vi "ACal-Create Weighted Stimulus.vi"(0 "Weighted":T3 {"WF" items=["Chirp", "Noise"]}, 5 "Cal Stimulus":T1, 7 "Speaker":T2, 11 "error in (no error)":errorcluster) -> (4 "Stimulus":dbl[](array[numeric]), 15 "error out":errorcluster)   [LabVIEW 2020]
uses:
  Type Defs/ACal-Multiband Parameters.ctl
  epl-vi-lib/Utility VIs/Type Defs/Speaker ring.ctl
  Type Defs/Cal Stimulus.ctl
  Inverse Filter VIs/InvFilt-Params.ctl
  epl-vi-lib/Utility VIs/Math VIs/dB to Linear (scalar).vi
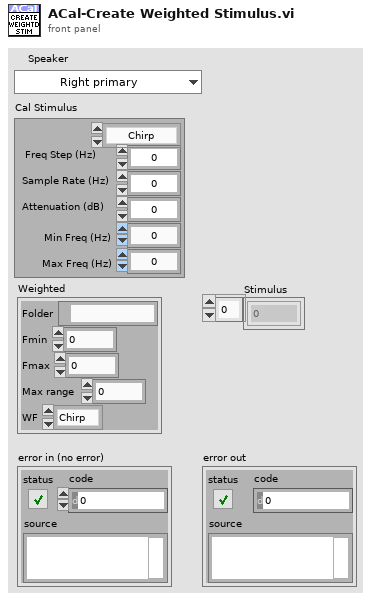
[diagram p1: front panel]
types:
  T1 = typedef "Cal Stimulus.ctl" = cluster{"Min Freq (Hz)":dbl, "Max Freq (Hz)":dbl, "Freq Step (Hz)":dbl, "Waveform":enum16{"Chirp", "Weighted"}, "Attenuation (dB)":dbl, "Sample Rate (Hz)":dbl}
  T2 = typedef "Speaker ring.ctl" = enum16{"Right primary", "Right secondary", "Left primary", "Left secondary"}
  T3 = typedef "ACal-Multiband Parameters.ctl" = cluster{"Folder":path, "Fmin":dbl, "Fmax":dbl, "Max range":dbl, "WF":u16}
  T4 = typedef "InvFilt-Params.ctl" = cluster{"Min Frequency (Hz)":dbl, "Max Frequency (Hz)":dbl, "Length (points)":i32, "Sampling rate (Hz)":dbl, "Delay (ms)":dbl, "Linear phase":bool}
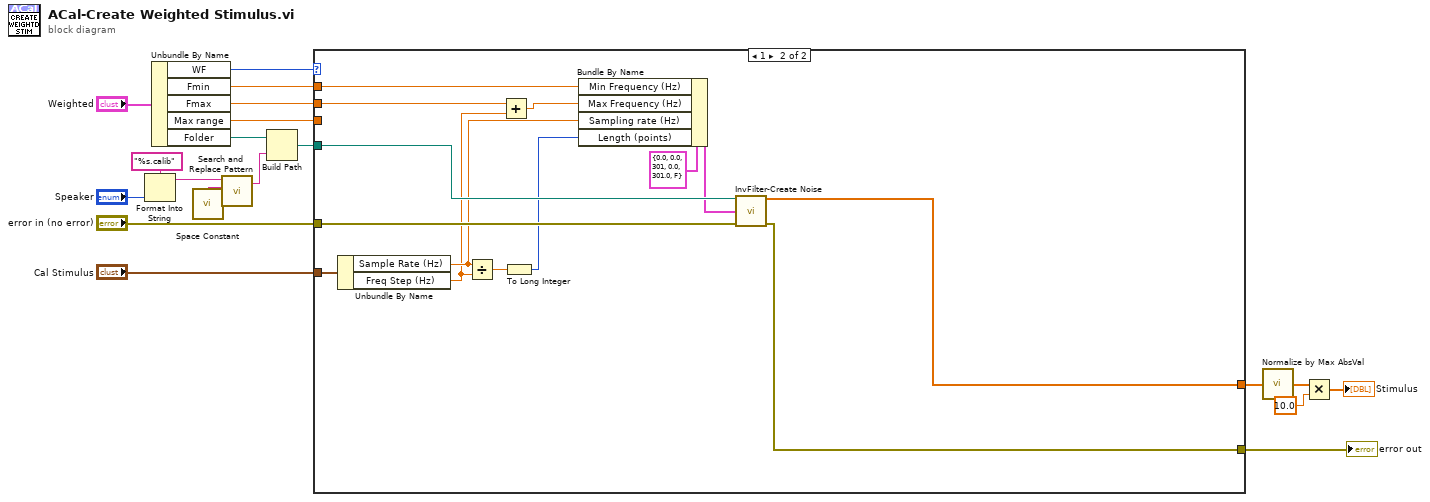
[diagram p0: block diagram]
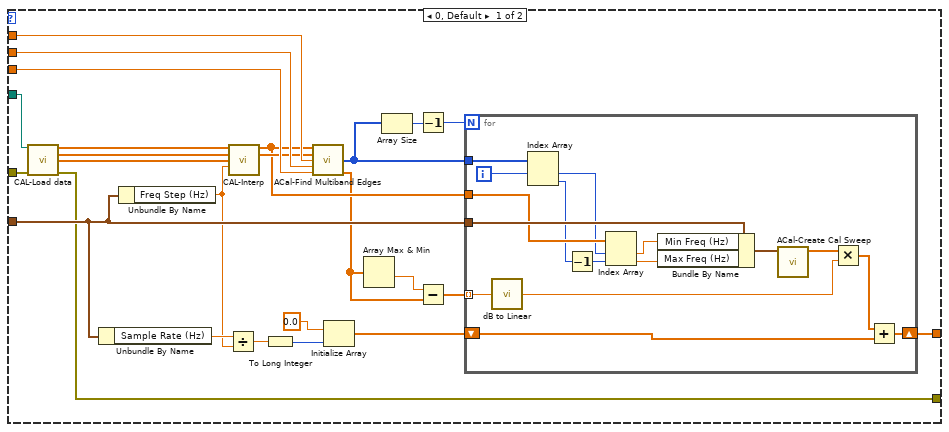
[diagram p2: hidden frame]
diagram:
  n1 = Format Into String(format string="%s.calib", "Speaker") -> (resulting string=w9:string)  [unwired: 2 in, 1 out]
  n2 = Unbundle By Name("Weighted") -> ("WF"=w5:u16, "Fmin"=w12:dbl, "Fmax"=w13:dbl, "Max range"=w14:dbl, "Folder"=w18:path)
  n3 = call <vilib>:"Space Constant.vi"() -> ("String"=w7:string)
  n4 = call <vilib>:"Search and Replace Pattern.vi"("string"=w9, "regular expression (\"\")"=w7) -> ("result string"=w8:string)  [unwired: 3 in, 1 out]
  n5 = Build Path(base path=w18, name or relative path=w8) -> (appended path=w15:path)
  n6 = case shown="1" w5 {
    tunnel: w15 -> [w44 w74]
    tunnel: w14 -> [w43 _]
    tunnel: w13 -> [w42 w65]
    tunnel: w12 -> [w41 w66]
    tunnel: "error in (no error)" -> [w40 w70]
    tunnel: "Cal Stimulus" -> [w31 w71]
    tunnel: [w21 w69] -> w6
    tunnel: [w20 w68] -> w2
    frame 0, Default {
      n7 = call "CAL-Load data.vi"("user path"=w44, "error in (no error)"=w40) -> ("Frequency (Hz)"=w39:dbl[], "Mag"=w38:dbl[], "Phase"=w37:dbl[], "error out"=w21:errorcluster)  [unwired: 6 in, 4 out]
      n8 = Unbundle By Name(w31) -> ("Sample Rate (Hz)"=w30:dbl)
      n9 = Unbundle By Name(w31) -> ("Freq Step (Hz)"=w29:dbl)
      n10 = Divide(x=w30, y=w29) -> (x/y=w28:dbl)
      n11 = call "CAL-Interp.vi"("Frequency (Hz)"=w39, "Magnitude (dB)"=w38, "Phase (degrees)"=w37, "df (Hz)"=w29) -> ("Interp Freq (Hz)"=w35:dbl[], "Interp Magnitude (dB)"=w36:dbl[])  [unwired: 8 in, 2 out]
      n12 = To Long Integer(number=w28) -> (32bit integer=w27:i32)
      n13 = call "ACal-Find Multiband Edges.vi"("Freq"=w35, "Mag"=w36, "Fmin"=w41, "Fmax"=w42, "Max Range"=w43) -> ("Istart"=w34:i32[], "Mags"=w23:dbl[])  [unwired: 8 in, 1 out]
      n14 = Initialize Array(0.0, w27) -> (w25:dbl[])
      n15 = Array Max & Min(array=w23) -> (min value=w24:dbl)  [unwired: 3 out]
      n16 = Array Size(array=w34) -> (size(s)=w33:i32)
      n17 = Decrement(x=w33) -> (x-1=w32:i32)
      n18 = Subtract(x=w24, y=w23) -> (x-y=w22:dbl[])
      n19 = for {
        N: w32 -> [_]
        tunnel: w31 -> [w60]
        tunnel: w34 -> [w57]
        tunnel: w35 -> [w58]
        shift-right: [w48] -> w20
        shift-left: w25 -> [w49]
        tunnel: w22 -> [w47] mode=indexing
        i -> [w56]
        n20 = call-poly "dB to Linear.vi"("dB"=w47) -> ("linear"=w45:dbl)
        n21 = Index Array(array=w57, index #1=w56) -> (element #1=w55:i32, element #2=w54:i32)  [unwired: 1 in]
        n22 = Decrement(x=w54) -> (x-1=w51:i32)
        n23 = Index Array(array=w58, index #1=w55, index #2=w51) -> (element #1=w53:dbl, element #2=w52:dbl)
        n24 = Bundle By Name(cluster=w60, "Min Freq (Hz)"=w53, "Max Freq (Hz)"=w52) -> (w59:T1)
        n25 = call "ACal-Create Cal Sweep.vi"("Cal Stimulus"=w59) -> ("Stimulus"=w50:dbl[])  [unwired: 8 in, 2 out]
        n26 = Multiply(x=w50, y=w45) -> (x*y=w46:dbl[])
        n27 = Add(x=w46, y=w49) -> (x+y=w48:dbl[])
      }
    }
    frame 1 {
      n28 = Unbundle By Name(w71) -> ("Sample Rate (Hz)"=w64:dbl, "Freq Step (Hz)"=w61:dbl)
      n29 = Divide(x=w64, y=w61) -> (x/y=w72:dbl)
      n30 = Add(x=w65, y=w61) -> (x+y=w62:dbl)
      n31 = To Long Integer(number=w72) -> (32bit integer=w63:i32)
      n32 = Bundle By Name(cluster=T4 {"Min Frequency (Hz)"=0.0, "Max Frequency (Hz)"=0.0, "Length (points)"=301, "Sampling rate (Hz)"=0.0, "Delay (ms)"=301.0, "Linear phase"=FALSE} ("InvFilt Params"), "Min Frequency (Hz)"=w66, "Max Frequency (Hz)"=w62, "Sampling rate (Hz)"=w64, "Length (points)"=w63) -> (w67:T4)
      n33 = call "InvFilter-Create Noise.vi"("Calibration File"=w74, "InvFilt Params"=w67, "error in (no error)"=w70) -> ("InvFilter Noise"=w68:dbl[], "error out"=w69:errorcluster)  [unwired: 9 in, 2 out]
    }
  }
  "error out" <- w6
  n34 = call "Normalize by Max AbsVal.vi"("Y"=w2) -> ("Ynorm"=w3:dbl[])
  n35 = Multiply(x=w3, y=10.0) -> (x*y=→"Stimulus":dbl[])
